vi "Create Data File.vi"(8 "Error In":errorcluster) -> (0 "Error Out":errorcluster, 3 "File Refnum":refnum<file>)   [LabVIEW 2012]
doc: "This VI performs a series of tasks to create a file for logging data:\n\n1) Check to see if a folder called 'Logged Data' exsists in the same directory as the application\n2) If the folder does not exsist, create it\n3) Create a file name of the format 'Acquired Data <Date> <Time>.txt'\n4) Replace or Create the file"
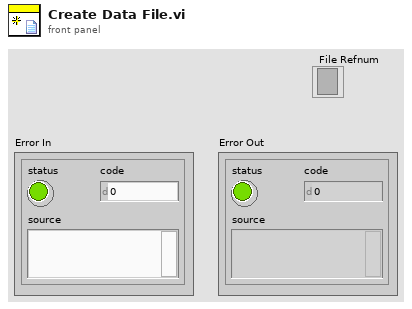
[diagram p1: front panel]
types:
  T1 = enum16{"open", "replace", "create", "open or create", "replace or create", "replace or create with confirmation"}
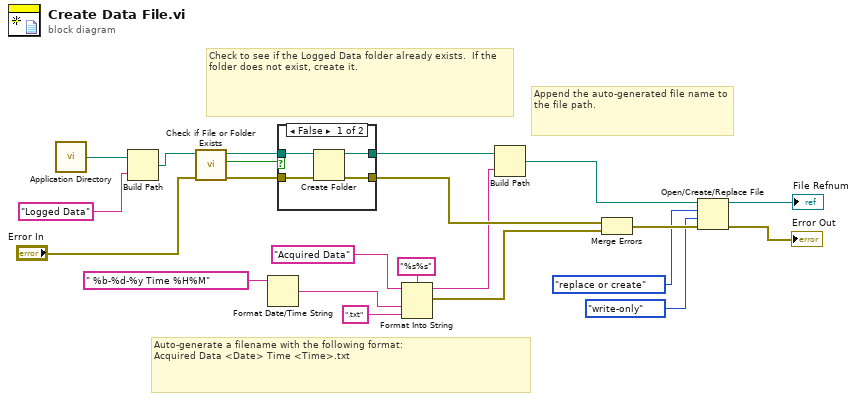
[diagram p0: block diagram]
diagram:
  # "Append the auto-generated file name to the file path."
  # "Check to see if the Logged Data folder already exists.  If the folder does not exist, create it."
  # "Auto-generate a filename with the following format:\nAcquired Data <Date> Time <Time>.txt"
  n1 = call <vilib>:"Application Directory.vi"() -> ("Application Directory"=w8:path)
  n2 = Build Path(base path=w8, name or relative path="Logged Data" ("prompt (Create Folder)")) -> (appended path=w12:path)
  n3 = call <vilib>:"Check if File or Folder Exists.vi"("error in (no error)"="Error In", "path"=w12) -> ("error out"=w11:errorcluster, "file or folder exists?"=w9:bool, "dup path"=w10:path)  [unwired: 7 in]
  n4 = Format Date/Time String(time format string (%c)=" %b-%d-%y Time %H%M") -> (date/time string=w4:string)  [unwired: 2 in]
  n5 = case shown="False" w9 {
    tunnel: [w26 w28] -> w15
    tunnel: [w25 w27] -> w14
    tunnel: w11 -> [w24 w27]
    tunnel: w10 -> [w23 w28]
    frame False {
      n6 = Create Folder(path (use dialog)=w23, error in=w24) -> (created path=w26:path, error out=w25:errorcluster)  [unwired: 1 in, 1 out]
    }
    frame True {
    }
  }
  n7 = Format Into String(format string="%s%s", initial string="Acquired Data" ("string"), w4, ".txt" ("string")) -> (resulting string=w1:string, error out=w2:errorcluster)  [unwired: 1 in]
  n8 = Build Path(base path=w15, name or relative path=w1) -> (appended path=w22:path)
  n9 = Merge Errors(w14, w2) -> (w21:errorcluster)
  n10 = Open/Create/Replace File(file path (use dialog)=w22, error in=w21, operation (0:open)=T1."replace or create", access (0:read/write)=enum16{"read/write", "read-only", "write-only"}."write-only") -> (refnum out=→"File Refnum":refnum<file>, error out=→"Error Out":errorcluster)  [unwired: 2 in, 1 out]
